vi "SendHeaderSD.vi"(8 "error in (no error)":errorcluster, 10 "Header":string, 11 "SerialPortRef":T1) -> (0 "error out":errorcluster, 3 "SerialPortRef 2":T1)   [LabVIEW 2016]
uses:
  <vilib>/Rock Robotics/WPI/SerialPort/WPI_SerialPortRef.ctl
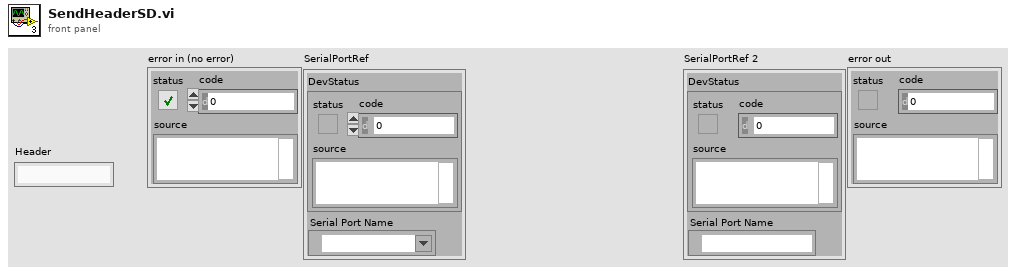
[diagram p1: front panel]
types:
  T1 = typedef "WPI_SerialPortRef.ctl" = cluster{"DevStatus":errorcluster, "Serial Port Name":refnum<visa-resource-name>}
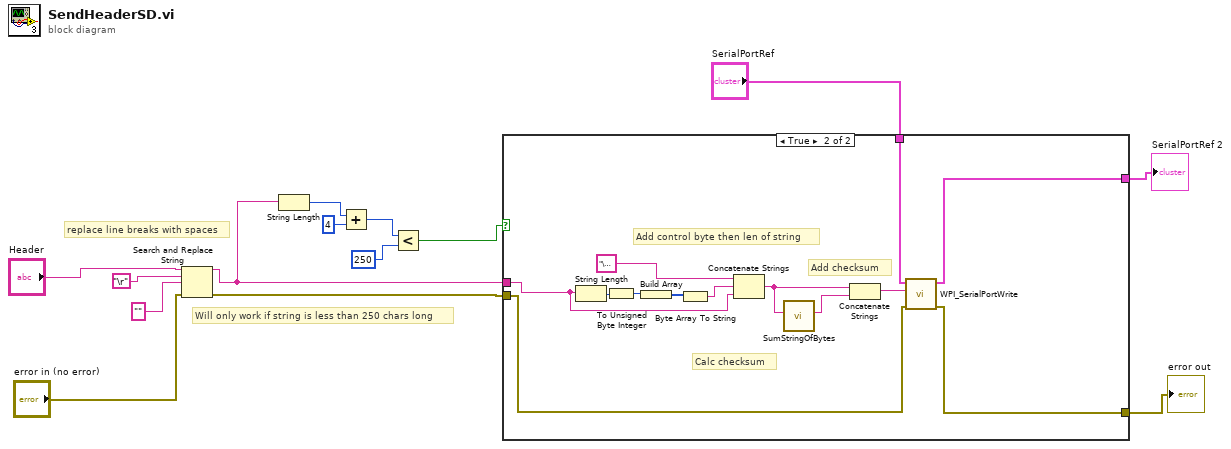
[diagram p0: block diagram]
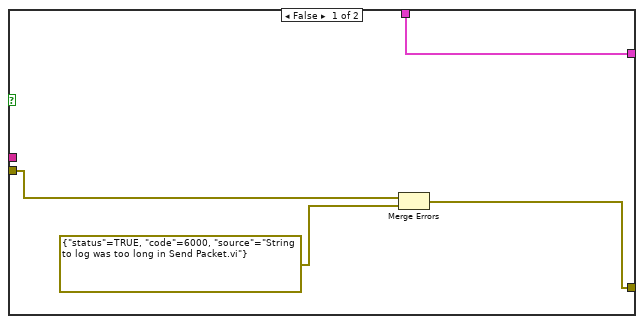
[diagram p2: hidden frame]
diagram:
  # "Will only work if string is less than 250 chars long"
  # "replace line breaks with spaces"
  n1 = Search and Replace String(input string="Header", search string="\r", replace string="" ("replace string (\"\")"), error in="error in (no error)") -> (result string=w4:string, error out=w8:errorcluster)  [unwired: 4 in, 2 out]
  n2 = String Length(string=w4) -> (length=w6:i32)
  n3 = Add(x=w6, y=4) -> (x+y=w10:i32)
  n4 = Less?(x=w10, y=250) -> (x < y?=w5:bool)
  n5 = case shown="True" w5 {
    tunnel: w8 -> [w18 w23]
    tunnel: w4 -> [_ w22]
    tunnel: "SerialPortRef" -> [w15 w21]
    tunnel: [w16 w20] -> w2
    tunnel: [w15 w19] -> w1
    frame False {
      n6 = Merge Errors(w18, errorcluster {"status"=TRUE, "code"=6000, "source"="String to log was too long in Send Packet.vi"} ("error out")) -> (w16:errorcluster)
    }
    frame True {
      # "Calc checksum"
      # "Add checksum"
      # "Add control byte then len of string"
      n7 = String Length(string=w22) -> (length=w30:i32)
      n8 = To Unsigned Byte Integer(number=w30) -> (unsigned 8bit integer=w27:u8)
      n9 = Build Array(w27) -> (w28:u8[])
      n10 = Byte Array To String(unsigned byte array=w28) -> (string=w29:string)
      n11 = Concatenate Strings("\u0002", w29, w22) -> (w25:string)
      n12 = call "SumStringOfBytes.vi"("String Of Bytes"=w25) -> ("SumAsString"=w24:string)  [unwired: 10 in]
      n13 = Concatenate Strings(w25, w24) -> (w31:string)
      n14 = call <vilib>:"WPI_SerialPortWrite.vi"("error in (no error)"=w23, "Buffer"=w31, "SerialPortRef"=w21) -> ("error out"=w20:errorcluster, "SerialPortRef"=w19:T1)  [unwired: 6 in, 1 out]
    }
  }
  "SerialPortRef 2" <- w1
  "error out" <- w2
